vi "累积列表-报警列表-XY曲线-内容.vi"(11 "绑定的数据":T8) -> (0 "时间范围":cluster{"max-x":timestamp, "min-x":timestamp}, 1 "报警列表内容":string[](array[string]), 2 "累积列表内容":string[](array[string]), 3 "XY图曲线数据":cluster{"数组":timestamp[], "数组":dbl[]}[](array[cluster]), 4 "数值范围":cluster{"max-y":dbl, "min-y":dbl})   [LabVIEW 2017]
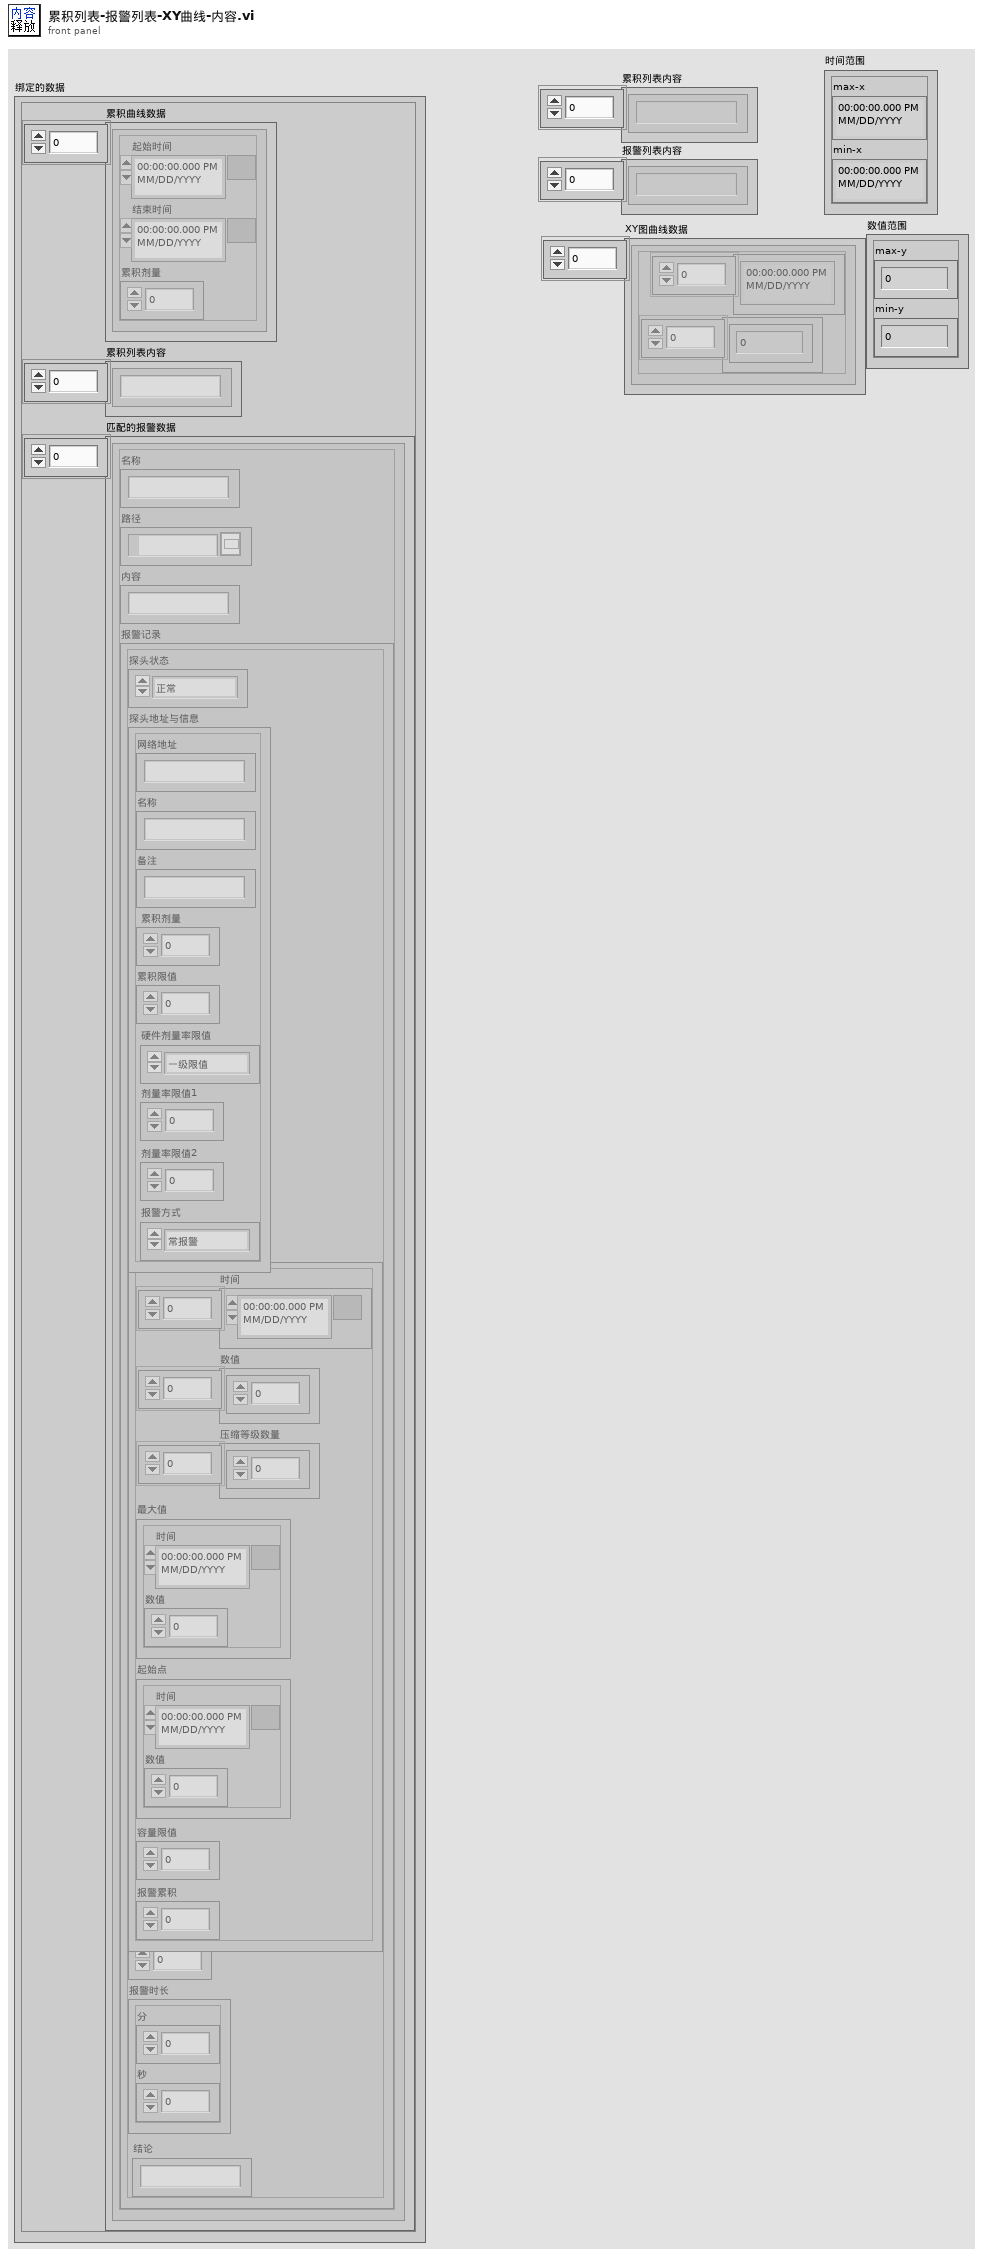
[diagram p1: front panel]
types:
  T1 = typedef "单条累积记录.ctl" = cluster{"起始时间":timestamp, "结束时间":timestamp, "累积剂量":dbl}
  T2 = typedef "通用报警记录.ctl" = cluster{"探头状态":T3, "探头地址与信息":T4, "缓存绘图数据":T7, "平均值":dbl, "报警时长":cluster{"分":u16, "秒":u16}, "结论":string}
  T3 = typedef "探头状态.ctl" = enum16{"正常", "离线", "禁用", "一级报警", "二级报警", "累积报警"}
  T4 = typedef "探测器信息.ctl" = cluster{"网络地址":string, "名称":string, "备注":string, "累积剂量":dbl, "累积限值":dbl, "硬件剂量率限值":T5, "剂量率限值1":dbl, "剂量率限值2":dbl, "报警方式":T6}
  T5 = typedef "探头剂量率限值选择.ctl" = enum16{"一级限值", "二级限值"}
  T6 = typedef "报警方式选择.ctl" = enum16{"常报警", "自动静音", "手动静音"}
  T7 = typedef "时值缓存压缩模块.lvlib/缓存数据.ctl" = cluster{"时间":timestamp[], "数值":dbl[], "压缩等级数量":i32[], "最大值":cluster{"时间":timestamp, "数值":dbl}, "起始点":cluster{"时间":timestamp, "数值":dbl}, "容量限值":i32, "报警累积":dbl}
  T8 = cluster{"累积曲线数据":T1[], "累积列表内容":string[], "匹配的报警数据":cluster{"名称":string, "路径":path, "内容":string, "报警记录":T2}[]}
  T9 = typedef "浏览XY图曲线索引.ctl" = enum16{"最大值-选中", "最大值点", "率警-选中", "率警", "累积-选中", "累积-超限", "累积"}
  T10 = cluster{"名称":string, "路径":path, "内容":string, "报警记录":T2}[]
  T11 = enum16{"绝对差值", "取整+1s", "取整+1m", "取整+1h", "取整+1d"}
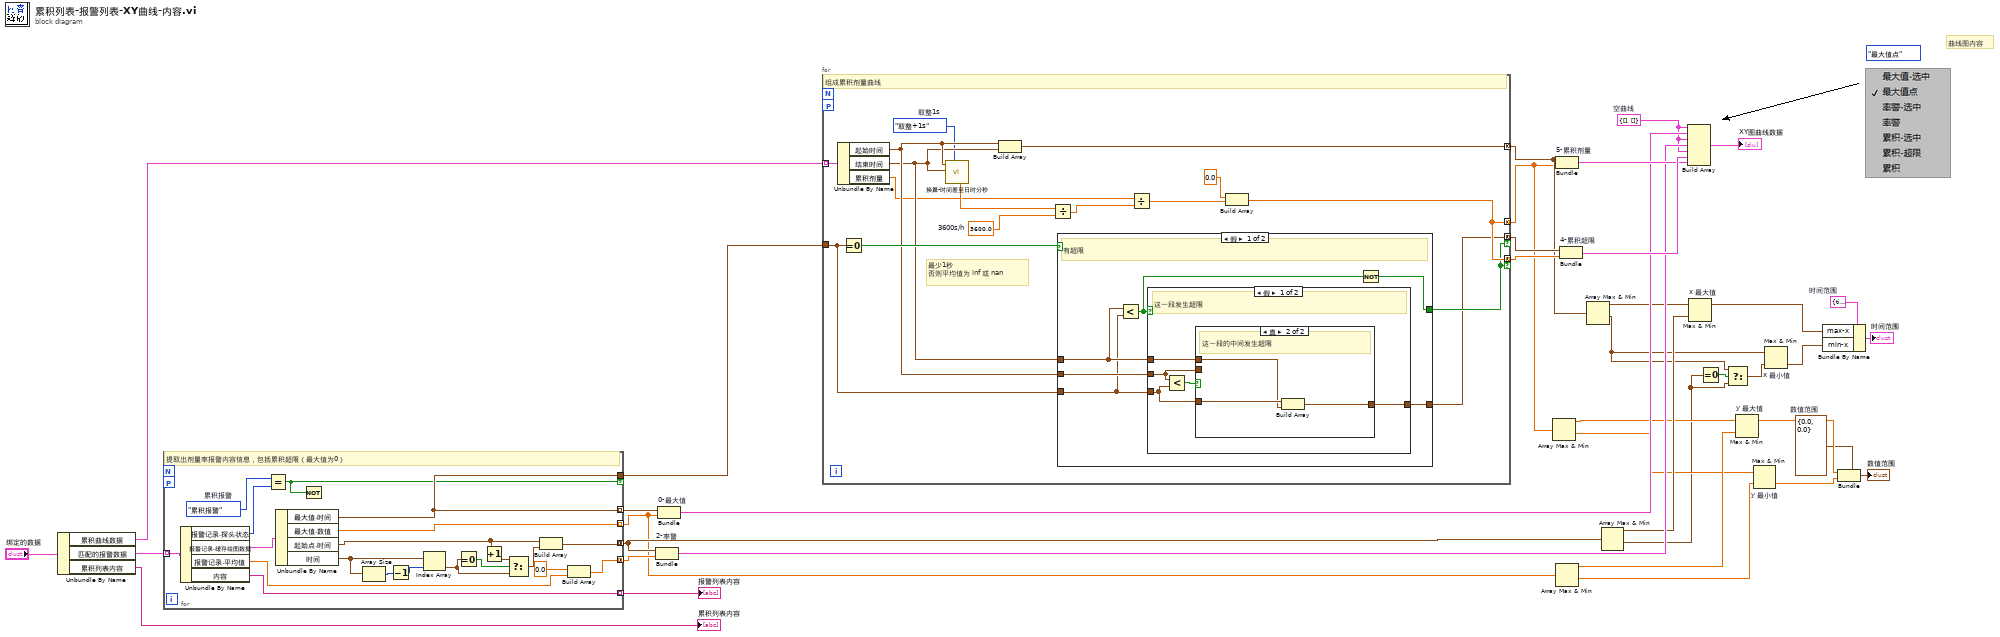
[diagram p0: block diagram]
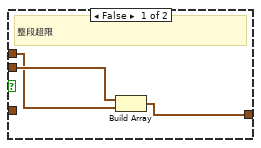
[diagram p2: hidden frame]
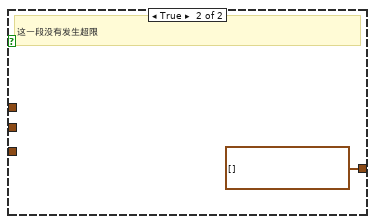
[diagram p3: hidden frame]
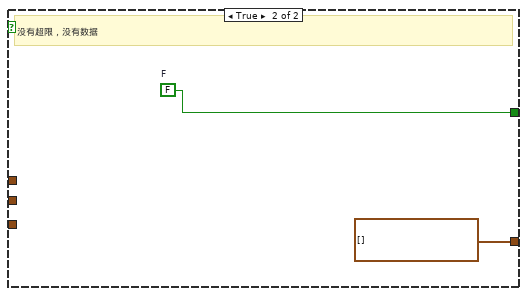
[diagram p4: hidden frame]
diagram:
  w7 = cluster{"max-y":dbl, "min-y":dbl} {"max-y"=0.0, "min-y"=0.0}  # 数值范围
  w17 = cluster{"max-x":timestamp, "min-x":timestamp} {"max-x"=timestamp(0 s since 1904-01-01), "min-x"=timestamp(0 s since 1904-01-01)}  # 时间范围
  (unwired) 浏览XY图曲线索引."最大值点" ("枚举")
  w24 = cluster{timestamp[], dbl[]} {[], []}  # 空曲线
  # "曲线图内容"
  n1 = Unbundle By Name("绑定的数据") -> ("累积曲线数据"=w30:T1[], "匹配的报警数据"=w34:T10, "累积列表内容"=→"累积列表内容":string[])
  n2 = for {
    tunnel: w34 -> [w48] mode=indexing
    tunnel: [w54] -> w26 mode=indexing
    workers-P: _ -> [_]
    tunnel: [w51] -> w22 mode=concatenating
    tunnel: [w50] -> w14 mode=concatenating
    tunnel: [w45] -> w29 mode=indexing
    tunnel: [w49] -> w5 mode=indexing
    tunnel: [w45] -> w38 if=w44
    w46 = 探头状态."累积报警"  # 累积报警
    # "提取出剂量率报警内容信息，包括累积超限（最大值为0）"
    n3 = Unbundle By Name(w48) -> ("报警记录.探头状态"=w47:T3, "报警记录.缓存绘图数据"=w58:T7, "报警记录.平均值"=w53:dbl, "内容"=w54:string)
    n4 = Equal?(x=w46, y=w47) -> (x = y?=w44:bool)
    n5 = Unbundle By Name ("按名称解除捆绑")(w58) -> ("最大值.时间"=w45:timestamp, "最大值.数值"=w49:dbl, "起始点.时间"=w42:timestamp, "时间"=w56:timestamp[])
    n6 = Not(x=w44) -> ()  [unwired: 1 out]
    n7 = Array Size(array=w56) -> (size(s)=w57:i32)
    n8 = Decrement(x=w57) -> (x-1=w55:i32)
    n9 = Index Array(array=w56, index=w55) -> (element=w39:timestamp)
    n10 = Equal To 0?(x=w39) -> (x = 0?=w43:bool)
    n11 = Increment(x=w42) -> (x+1=w41:timestamp)
    n12 = Select(t=w41, s=w43, f=w39) -> (s? t:f=w40:timestamp)
    n13 = Build Array(w42, w40) -> (w51:timestamp[])
    n14 = Build Array(0.0 ("元素"), w53) -> (w50:dbl[])
  }
  "报警列表内容" <- w26
  n15 = Bundle "2-率警"(w22, w14) -> (w32:cluster{timestamp[], dbl[]})  [unwired: 1 in]
  n16 = Bundle "0-最大值"(w29, w5) -> (w31:cluster{timestamp[], dbl[]})  [unwired: 1 in]
  n17 = for {
    tunnel: w30 -> [w74] mode=indexing
    tunnel: [w72] -> w23 mode=concatenating
    tunnel: [w71] -> w15 mode=concatenating
    tunnel: [w67] -> w35 mode=concatenating if=w69
    tunnel: [w71] -> w36 mode=concatenating if=w69
    workers-P: _ -> [_]
    tunnel: w38 -> [w68]
    w59 = T11."取整+1s"  # 取整1s
    w65 = 3600.0  # 3600s/h
    # "最少1秒\n否则平均值为 inf 或 nan"
    # "组成累积剂量曲线"
    n18 = Unbundle By Name(w74) -> ("起始时间"=w64:timestamp, "结束时间"=w63:timestamp, "累积剂量"=w62:dbl)
    n19 = Equal To 0?(x=w68) -> (x = 0?=w70:bool)
    n20 = call "换算-时间差至日时分秒.vi"("时长模式"=w59, "时间1"=w63, "时间2"=w64) -> ("时长 s"=w66:dbl)  [unwired: 7 in, 1 out]
    n21 = Build Array(w64, w63) -> (w72:timestamp[])
    n22 = Divide(x=w66, y=w65) -> (x/y=w60:dbl)
    n23 = case shown="假" w70 {
      tunnel: [w76 w94] -> w69
      tunnel: w68 -> [w78 _]
      tunnel: w63 -> [w79 _]
      tunnel: w64 -> [w80 _]
      tunnel: [w75 timestamp[] []] -> w67
      frame False {
        # "有超限"
        n24 = Less?(x=w79, y=w78) -> (x < y?=w77:bool)
        n25 = case shown="假" w77 {
          tunnel: w78 -> [w84 _]
          tunnel: w79 -> [w83 _]
          tunnel: w80 -> [w82 _]
          tunnel: [w81 timestamp[] []] -> w75
          frame False {
            # "这一段发生超限"
            n26 = Less?(x=w82, y=w84) -> (x < y?=w85:bool)
            n27 = case shown="真" w85 {
              tunnel: w84 -> [_ w91]
              tunnel: w83 -> [w87 w90]
              tunnel: w82 -> [w88 _]
              tunnel: [w86 w89] -> w81
              frame False {
                # "整段超限"
                n28 = Build Array(w88, w87) -> (w86:timestamp[])
              }
              frame True {
                # "这一段的中间发生超限"
                n29 = Build Array(w91, w90) -> (w89:timestamp[])
              }
            }
          }
          frame True {
            # "这一段没有发生超限"
          }
        }
        n30 = Not(x=w77) -> (.not. x?=w76:bool)
      }
      frame True {
        w94 = FALSE  # F
        # "没有超限，没有数据"
      }
    }
    n31 = Divide(x=w62, y=w60) -> (x/y=w61:dbl)
    n32 = Build Array(0.0 ("元素"), w61) -> (w71:dbl[])
  }
  n33 = Array Max & Min(array=w15) -> (max value=w13:dbl, min value=w11:dbl)  [unwired: 2 out]
  n34 = Bundle "5-累积剂量"(w23, w15) -> (w33:cluster{timestamp[], dbl[]})  [unwired: 1 in]
  n35 = Array Max & Min(array=w5) -> (max value=w12:dbl, min value=w10:dbl)  [unwired: 2 out]
  n36 = Bundle "4-累积超限"(w35, w36) -> (w37:cluster{timestamp[], dbl[]})  [unwired: 1 in]
  n37 = Array Max & Min(array=w23) -> (max value=w21:timestamp, min value=w2:timestamp)  [unwired: 2 out]
  n38 = Array Max & Min(array=w22) -> (max value=w20:timestamp, min value=w1:timestamp)  [unwired: 2 out]
  n39 = Build Array(w24, w31, w24, w32, w24, w37, w33) -> (→"XY图曲线数据":cluster{timestamp[], dbl[]}[])
  n40 = Max & Min "x 最大值"(x=w21, y=w20) -> (max(x,y)=w19:timestamp)  [unwired: 1 out]
  n41 = Equal To 0?(x=w1) -> (x = 0?=w4:bool)
  n42 = Select(t=w2, s=w4, f=w1) -> (s? t:f=w3:timestamp)
  n43 = Max & Min "y 最大值"(x=w13, y=w12) -> (max(x,y)=w9:dbl)  [unwired: 1 out]
  n44 = Max & Min "y 最小值"(x=w11, y=w10) -> (min(x,y)=w8:dbl)  [unwired: 1 out]
  n45 = Max & Min "x 最小值"(x=w2, y=w3) -> (min(x,y)=w18:timestamp)  [unwired: 1 out]
  n46 = Bundle By Name(cluster=w17, "max-x"=w19, "min-x"=w18) -> (→"时间范围":cluster{"max-x":timestamp, "min-x":timestamp})
  n47 = Bundle(cluster=w7, "max-y"=w9, "min-y"=w8) -> (→"数值范围":cluster{"max-y":dbl, "min-y":dbl})
